vi "0-9 only.vi"(8 "error in (no error)":errorcluster, 9 "Numeric":u16) -> (0 "error out":errorcluster, 1 "String 2":string)   [LabVIEW 2023]
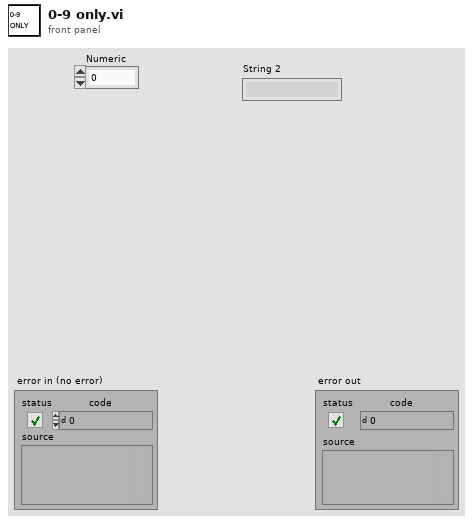
[diagram p1: front panel]
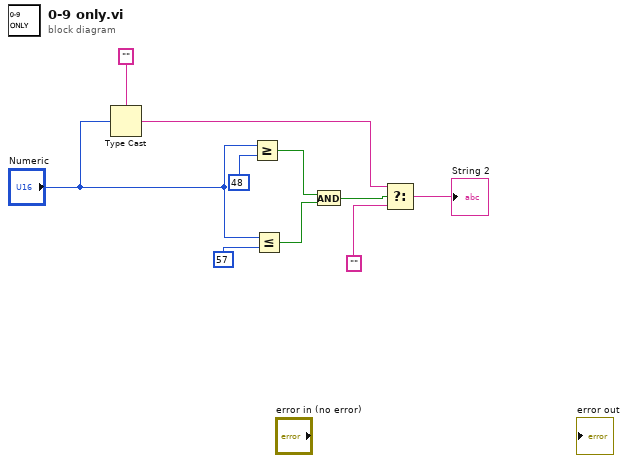
[diagram p0: block diagram]
diagram:
  n1 = Type Cast(type="", x="Numeric") -> (*(type *) &x=w3:string)
  n2 = Greater Or Equal?(x="Numeric", y=u8 48) -> (x >= y?=w8:bool)
  n3 = Less Or Equal?(x="Numeric", y=u8 57) -> (x <= y?=w7:bool)
  n4 = And(x=w8, y=w7) -> (x .and. y?=w6:bool)
  n5 = Select(t=w3, s=w6, f="") -> (s? t:f=→"String 2":string)
